vi "Acquire-single-image.vi"(8 "error in (no error)":errorcluster, 9 "Trigger ok?":bool, 10 "Images in":T1[](array[typedef]), 11 "Config. params. ref. in":refnum<data-value>) -> (0 "error out":errorcluster, 1 "Image ok?":bool, 2 "Images":T1[](array[typedef]), 3 "Config. params. ref.":refnum<data-value>)   [LabVIEW 2013, in "CameraVision.lvlib" / "CV-Acquisition.lvclass"]
uses:
  CV-Acquisition.lvclass
  Configuration/CV-Configuration.lvclass
  <vilib>/vision/Image Controls.llb/IMAQ Image.ctl
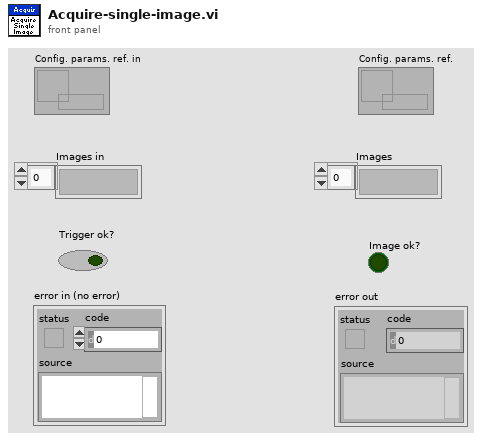
[diagram p1: front panel]
types:
  T1 = typedef "IMAQ Image.ctl" = refnum<image>
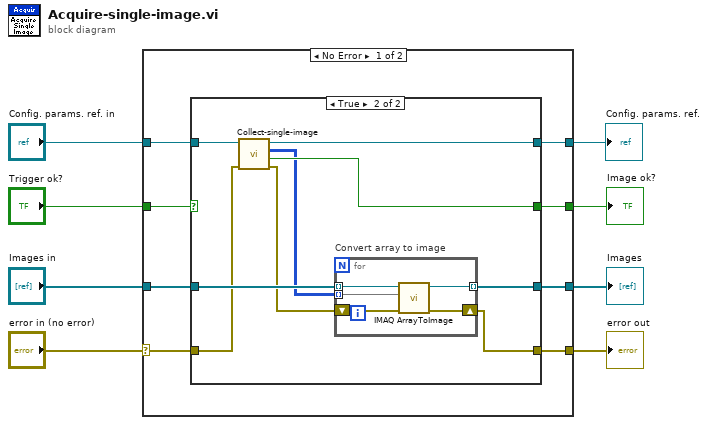
[diagram p0: block diagram]
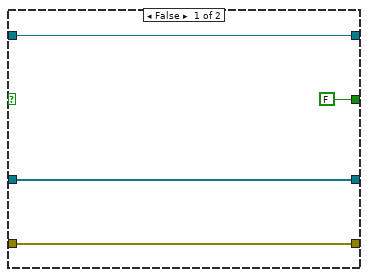
[diagram p2: hidden frame]
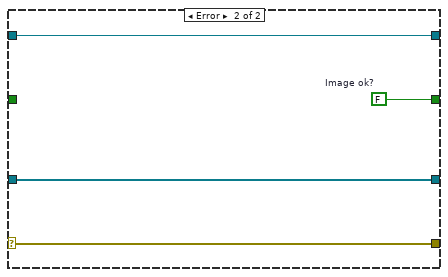
[diagram p3: hidden frame]
diagram:
  n1 = case shown="No Error" "error in (no error)" {
    selector: "error in (no error)" -> [w14 w38]
    tunnel: [w12 w38] -> w7
    tunnel: [w11 w37] -> w5
    tunnel: "Config. params. ref. in" -> [w15 w37]
    tunnel: "Images in" -> [w16 w36]
    tunnel: [w13 w36] -> w3
    tunnel: [w10 w35] -> w2
    tunnel: "Trigger ok?" -> [w9 _]
    frame No Error {
      n2 = case shown="True" w9 {
        tunnel: w16 -> [w18 w29]
        tunnel: w15 -> [w19 w28]
        tunnel: w14 -> [w17 w27]
        tunnel: [w18 w26] -> w13
        tunnel: [w17 w25] -> w12
        tunnel: [w19 w24] -> w11
        tunnel: [FALSE ("Image ok?") w23] -> w10
        frame False {
        }
        frame True {
          n3 = call "Collect-single-image.vi"("error in (no error)"=w27, "Config. params. ref. in"=w28) -> ("error out"=w21:errorcluster, "Image ok?"=w23:bool, "Images array"=w22:u8[][][], "Config. params. ref."=w24:refnum<data-value>)  [unwired: 6 in]
          n4 = for "Convert array to image" {
            tunnel: w29 -> [w34] mode=indexing
            tunnel: w22 -> [w33] mode=indexing
            shift-right: [w31] -> w25
            shift-left: w21 -> [w32]
            tunnel: [w30] -> w26 mode=indexing
            n5 = call "IMAQ ArrayToImage"("error in (no error)"=w32, "Image Pixels (U8)"=w33, "Image"=w34) -> ("error out"=w31:errorcluster, "Image Out"=w30:T1)  [unwired: 7 in]
          }
        }
      }
    }
    frame Error {
      w35 = FALSE  # Image ok?
    }
  }
  "error out" <- w7
  "Config. params. ref." <- w5
  "Images" <- w3
  "Image ok?" <- w2
